vi "main_fp.vi"() -> ()   [LabVIEW 2016]
uses:
  <vilib>/Instr/_visa.llb/Select Event Type.ctl
panel:
  in  "Tab Control":enum32{"Page 1"}(tab)
  out "Status of sensors":T1
  out "Waveform Chart":T2(graph)
  in  "VISA resource name":refnum<visa-resource-name>
  out "Internet OK":bool
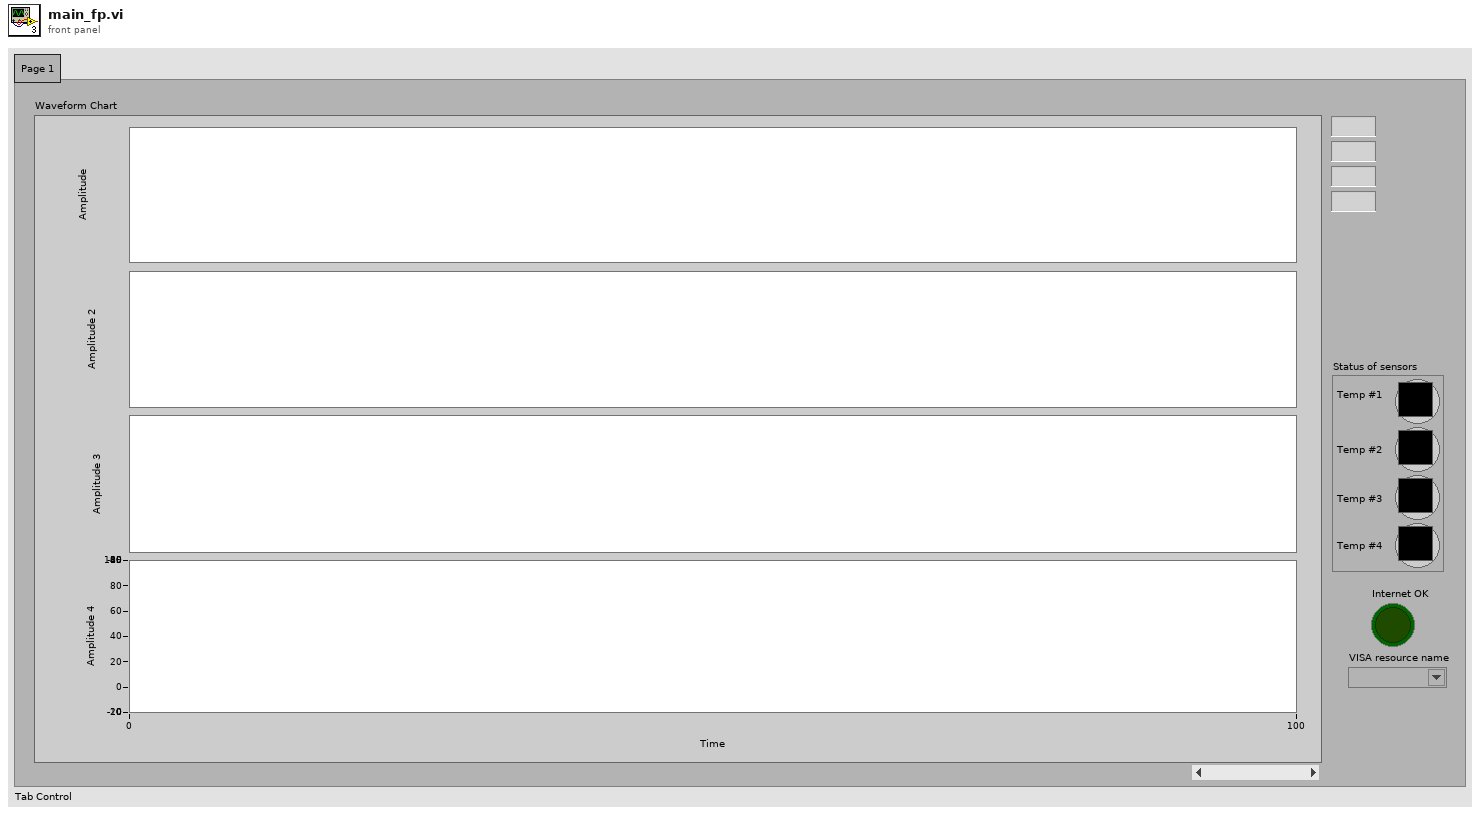
[diagram p1: front panel]
types:
  T1 = cluster{"Temp #1":u32, "Temp #2":u32, "Temp #3":u32, "Temp #4":u32}
  T2 = cluster{"[0]":dbl, "[1]":dbl, "[2]":dbl, "[3]":dbl}
  T3 = typedef "Select Event Type.ctl" = u32
  T4 = cluster{"[0]":u32, "[1]":u32, "[2]":u32, "[3]":u32}
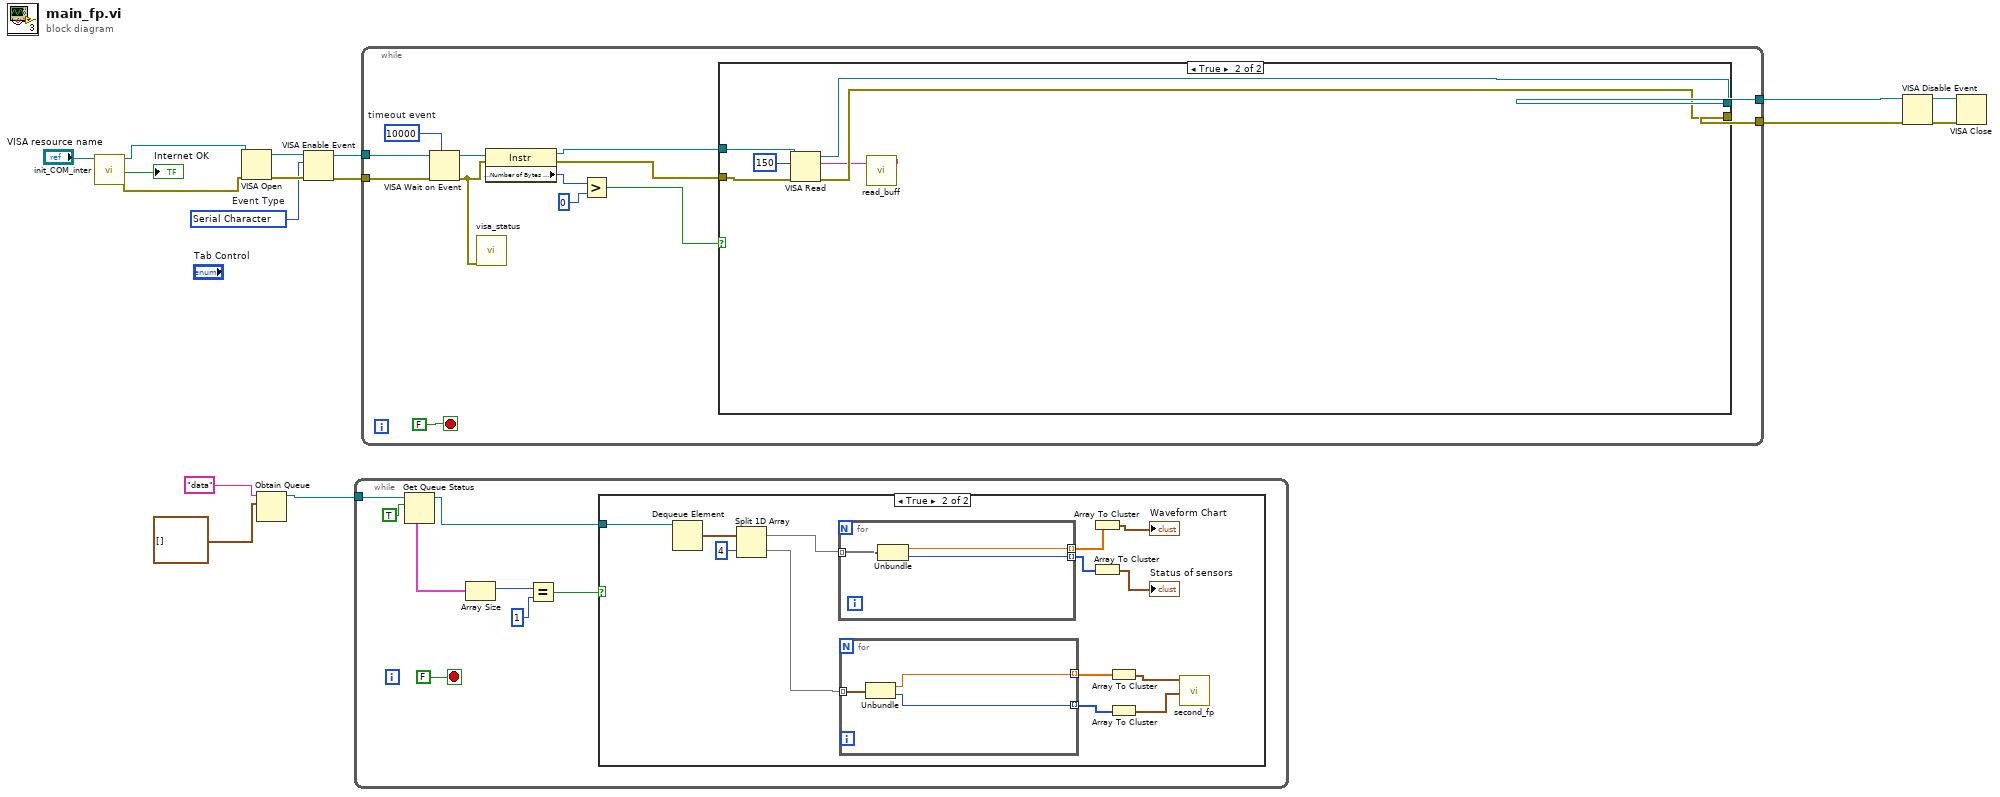
[diagram p0: block diagram]
diagram:
  w10 = T3 1073684533 items=["Service Request"=1073684491, "Trigger"=3221168138, "Clear"=1073684493, "VXI Signal"=1073684512, "VXI/VME Interrupt"=3221168161, "VXI/VME Sysfail"=1073684509, "VXI/VME Sysreset"=1073684510, "GPIB CIC"=1073684498, "GPIB Talk"=1073684499, "GPIB Listen"=1073684500, "PXI Interrupt"=1073684514, "Serial Break"=1073684515, "Serial TermChar"=1073684516, "Serial CTS"=1073684521, "Serial DSR"=1073684522, "Serial DCD"=1073684524, "Serial RI"=1073684526, "Serial Character"=1073684533, "USB Interrupt"=1073684535, "All Enabled"=1073709055]  # Event Type
  n1 = call "init_COM_inter.vi"("VISA Refnum in"="VISA resource name") -> ("VISA out"=w5:refnum<visa-resource-name>, "Internet OK"=→"Internet OK":bool, "VISA error out"=w4:errorcluster)  [unwired: 15 in, 1 out]
  n2 = VISA Open(error in (no error)=w4, VISA resource name=w5) -> (VISA resource name=w16:refnum<visa-resource-name>, error out=w15:errorcluster)  [unwired: 3 in]
  n3 = Obtain Queue(name (unnamed)="data", element data type=cluster{dbl, "Round Color Box":u32}[] []) -> (queue out=w1:refnum<queue>)  [unwired: 3 in, 2 out]
  n4 = VISA Enable Event(8:w15, 10:w10, 11:w16) -> (0:w13:errorcluster, 3:w14:refnum<visa-resource-name>)  [unwired: 1 in]
  n5 = while {
    tunnel: w1 -> [w23]
    stop <- FALSE stop-if-true
    n6 = Get Queue Status(queue=w23, return elements? (F)=TRUE) -> (queue out=w17:refnum<queue>, elements=w20:cluster{cluster{dbl, "Round Color Box":u32}[]}[])  [unwired: 1 in, 6 out]
    n7 = Array Size(array=w20) -> (size(s)=w21:i32)
    n8 = Equal?(x=w21, y=1) -> (x = y?=w18:bool)
    n9 = case shown="True" w18 {
      tunnel: w17 -> [_ w37]
      frame False {
      }
      frame True {
        n10 = Dequeue Element(queue=w37) -> (element=w36:cluster{dbl, "Round Color Box":u32}[])  [unwired: 2 in, 3 out]
        n11 = Split 1D Array(array=w36, index=4) -> (first subarray=w34:cluster{dbl, "Round Color Box":u32}[], second subarray=w33:cluster{dbl, "Round Color Box":u32}[])
        n12 = for {
          tunnel: w34 -> [w43] mode=indexing
          tunnel: [w42] -> w31 mode=indexing
          tunnel: [w41] -> w32 mode=indexing
          n13 = Unbundle(w43) -> (w41:dbl, "Round Color Box"=w42:u32)
        }
        n14 = for {
          tunnel: w33 -> [w40] mode=indexing
          tunnel: [w39] -> w30 mode=indexing
          tunnel: [w38] -> w29 mode=indexing
          n15 = Unbundle(w40) -> (w39:dbl, "Round Color Box"=w38:u32)
        }
        n16 = Array To Cluster(array=w32) -> (cluster=→"Waveform Chart":T2)
        n17 = Array To Cluster(array=w31) -> (cluster=→"Status of sensors":T4)
        n18 = Array To Cluster(array=w30) -> (cluster=w28:T2)
        n19 = Array To Cluster(array=w29) -> (cluster=w27:T4)
        n20 = call "second_fp.vi"("Waveform chart data"=w28, "Stat of sensors"=w27) -> ()  [unwired: 18 in]
      }
    }
  }
  n21 = while {
    tunnel: w14 -> [w56]
    tunnel: w13 -> [w48]
    tunnel: [w46] -> w9
    tunnel: [w45] -> w8
    stop <- FALSE stop-if-true
    w49 = u32 10000  # timeout event
    n22 = VISA Wait on Event(7:w49, 8:w48, 11:w56) -> (0:w47:errorcluster, 3:w55:refnum<visa-resource-name>)  [unwired: 2 in, 2 out]
    n23 = call "visa_status.vi"("error in (no error)"=w47) -> ()  [unwired: 11 in]
    n24 = property class="Instr"(reference=w55, error in=w47) -> (reference out=w54:refnum<visa-resource-name>, error out=w50:errorcluster, "Serial Settings:Number of Bytes at Serial Port"=w53:u32)
    n25 = Greater?(x=w53, y=u32 0) -> (0:w51:bool)
    n26 = case shown="True" w51 {
      tunnel: w54 -> [w58 w63]
      tunnel: w50 -> [w57 w62]
      tunnel: [w58 w61] -> w46
      tunnel: [w57 w60] -> w45
      frame False {
      }
      frame True {
        n27 = VISA Read(VISA resource name=w63, byte count=u32 150, error in (no error)=w62) -> (VISA resource name out=w61:refnum<visa-resource-name>, read buffer=w59:string, error out=w60:errorcluster)  [unwired: 1 out]
        n28 = call "read_buff.vi"("buffer"=w59) -> ()  [unwired: 9 in]
      }
    }
  }
  n29 = VISA Disable Event(8:w8, 11:w9) -> (0:w12:errorcluster, 3:w11:refnum<visa-resource-name>)  [unwired: 2 in]
  n30 = VISA Close(VISA resource name=w11, error in (no error)=w12) -> ()  [unwired: 1 out]
